vi "Edit_bad_calibration_coeff.vi"() -> ()   [LabVIEW 2010]
uses:
  Anemometry Sub Vis/Controls/File_Selector_Type.ctl
  Anemometry Sub Vis/Globals/Meas_global.vi
panel:
  out "index of element":i32
  out "bkgnd":string
  in  "Previous Choice":path
  in  "Search String":string
  in  "Boolean":bool
  in  "Pause Mode":enum16{"Continuous Running", "After Each File"}(ring)
  in  "At Dialog Prompt Post Process":T1
  out "Files Processed":i32(slide) scale=0.0..1.0
  in  "stop":bool
  out "Files To Process":path[](array[path])
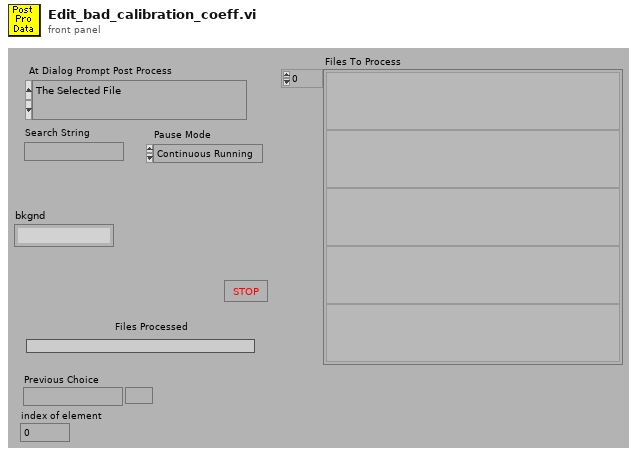
[diagram p1: front panel]
types:
  T1 = typedef "File_Selector_Type.ctl" = enum16{"The Selected File", "The Selected Folder", "Files containing the search string in the selected folder", "All files listed in selected file"}
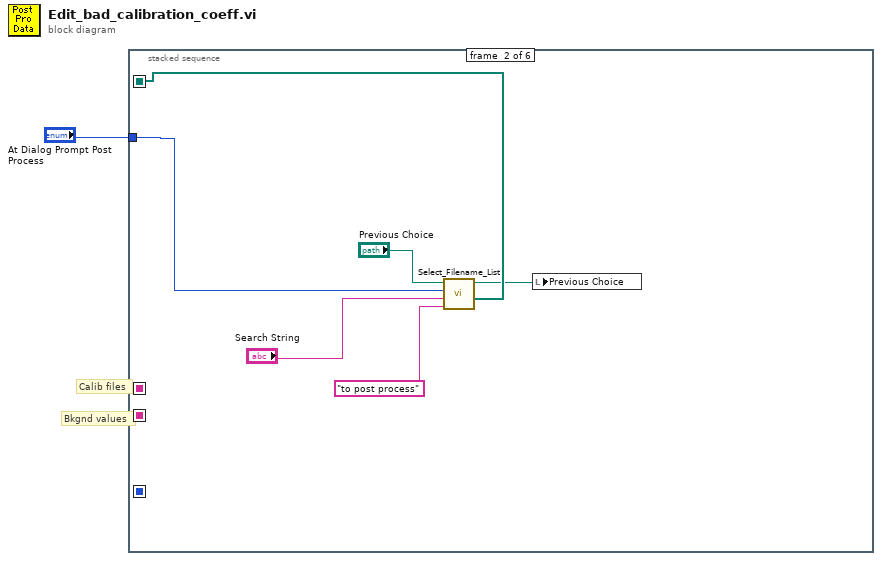
[diagram p0: block diagram]
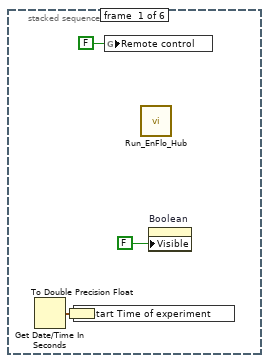
[diagram p2: hidden frame]
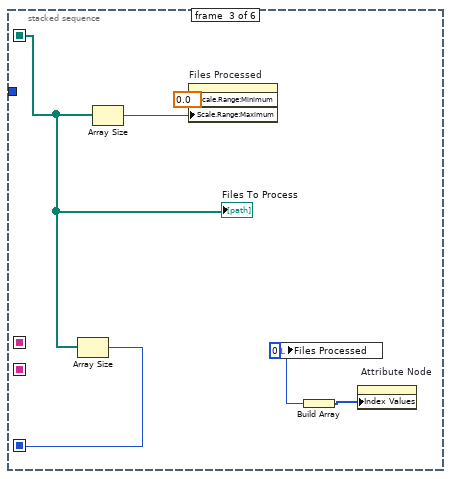
[diagram p3: hidden frame]
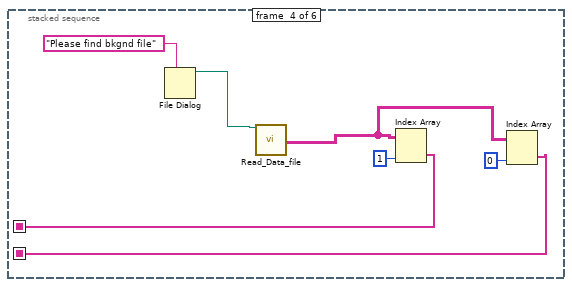
[diagram p4: hidden frame]
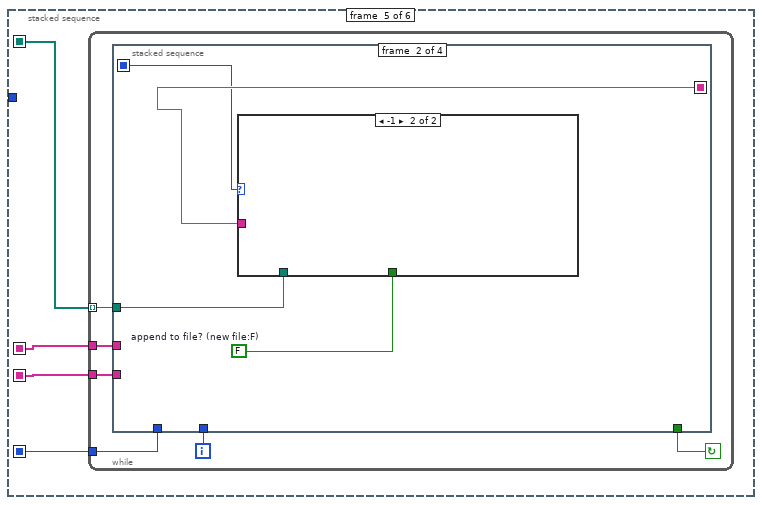
[diagram p5: hidden frame]
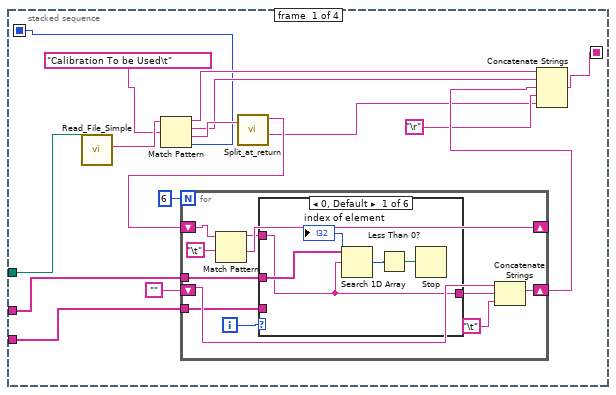
[diagram p6: hidden frame]
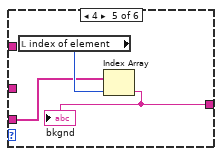
[diagram p10: hidden frame]
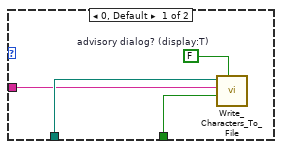
[diagram p12: hidden frame]
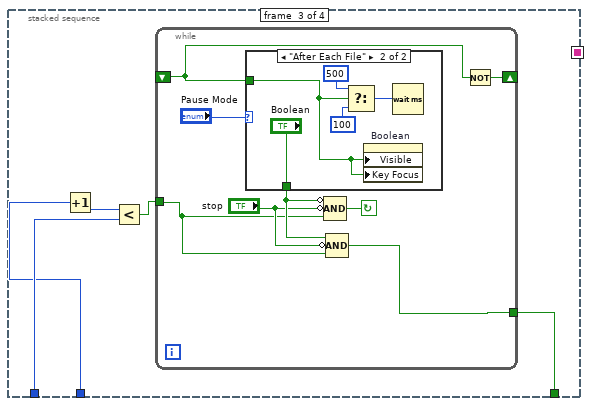
[diagram p13: hidden frame]
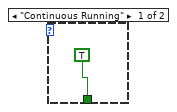
[diagram p14: hidden frame]
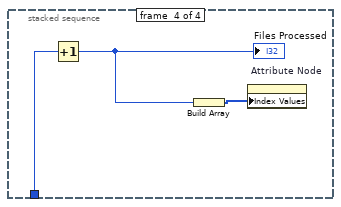
[diagram p15: hidden frame]
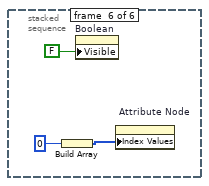
[diagram p16: hidden frame]
diagram:
  # "Bkgnd values"
  # "Calib files"
  n1 = stacked-sequence {
    seq-local: [_ _ w17 _ _ _] -> [_ _ _ _ w28 _]
    seq-local: [_ w10 _ _ _ _] -> [_ _ w12 _ w27 _]
    seq-local: [_ _ _ w21 _ _] -> [_ _ _ _ w26 _]
    seq-local: [_ _ _ w18 _ _] -> [_ _ _ _ w25 _]
    tunnel: "At Dialog Prompt Post Process" -> [_ w11 _ _ _ _]
    frame #0 {
      n2 = Get Date/Time In Seconds() -> (seconds since 1Jan1904=w2:timestamp)
      n3 = To Double Precision Float(number=w2) -> (double precision float=w3:dbl)
      n4 = global write "Meas_global.vi" "Start Time of experiment"(w3) -> ()
      n5 = global write "Meas_global.vi" "Remote control"(FALSE ("Remote control")) -> ()
      n6 = call "Run_EnFlo_Hub.vi"() -> ()  [unwired: 8 in]
      n7 = property on="Boolean" class="Bool"("Visible"=FALSE ("Write Attribute")) -> ()  [unwired: 2 in, 2 out]
    }
    frame #1 {
      n8 = call "Select_Filename_List.vi"("File Type"="to post process", "Search String"="Search String", "At Dialog Prompt Post Process"=w11, "Previous Choice"="Previous Choice") -> ("Selected files"=w10:path[], "Choosen path"=w6:path)  [unwired: 2 in, 1 out]
      n9 = local write "Previous Choice"(w6) -> ()
    }
    frame #2 {
      w13 = 0 ("Files Processed")
      n10 = Array Size(array=w12) -> (size(s)=w17:i32)
      n11 = Array Size(array=w12) -> (size(s)=w15:i32)
      n12 = property on="Files Processed" class="Slide (strict)"("Scale.Range:Minimum"=0.0 ("Write Attribute"), "Scale.Range:Maximum"=w15) -> ()  [unwired: 2 in, 2 out]
      n13 = local write "Files Processed"(w13) -> ()
      n14 = Build Array(w13) -> (w14:i32[])
      n15 = property on="Attribute Node" class="Arr (strict)"("Index Values"=w14) -> ()  [unwired: 2 in, 2 out]
      "Files To Process" <- w12
    }
    frame #3 {
      n16 = File Dialog(7:"Please find bkgnd file" ("prompt")) -> (3:w23:path)  [unwired: 6 in, 3 out]
      n17 = call "Read_Data_file.vi"("Results file"=w23) -> ("Channel Values Out"=w19:string[][])  [unwired: 9 in, 9 out]
      n18 = Index Array(array=w19, index (col)=1 ("disabled index (col)")) -> (element=w21:string[])  [unwired: 1 in]
      n19 = Index Array(array=w19, index (col)=0 ("disabled index (col)")) -> (element=w18:string[])  [unwired: 1 in]
    }
    frame #4 {
      n20 = while {
        tunnel: w27 -> [w31] mode=indexing
        tunnel: w28 -> [w34]
        tunnel: w26 -> [w30]
        tunnel: w25 -> [w29]
        i -> [w33]
        stop <- w32 continue-if-true
        n21 = stacked-sequence {
          seq-local: [w40 _ _ _] -> [_ w74 _ _]
          seq-local: [w35 _ _ _] -> [_ w73 _ _]
          tunnel: w31 -> [w50 w76 _ _]
          tunnel: w34 -> [_ _ w83 _]
          tunnel: w33 -> [_ _ w82 w101]
          tunnel: [_ _ w81 _] -> w32
          tunnel: w30 -> [w37 _ _ _]
          tunnel: w29 -> [w36 _ _ _]
          frame #0 {
            n22 = call "Read_File_Simple.vi"("Filename"=w50) -> ("string"=w47:string)  [unwired: 4 in, 5 out]
            n23 = Match Pattern(string=w47, regular expression="Calibration To be Used\t" ("Variable name")) -> (before substring=w43:string, match substring=w42:string, after substring=w45:string, offset past match=w35:i32)  [unwired: 1 in]
            n24 = call "Split_at_return.vi"("String"=w45) -> ("before substring"=w44:string, "after substring"=w38:string)  [unwired: 1 in, 2 out]
            n25 = for {
              N: 6 -> [_]
              shift-right: [w55] -> _
              shift-left: w44 -> [w60]
              shift-right: [w56] -> w41
              shift-left: "" -> [w58]
              tunnel: w37 -> [w52]
              tunnel: w36 -> [w51]
              i -> [w59]
              n26 = Match Pattern(string=w60, regular expression="\t") -> (before substring=w53:string, after substring=w55:string)  [unwired: 1 in, 2 out]
              n27 = case shown="0, Default" w59 {
                tunnel: [w64 w66 w67 w68 w69 w72] -> w54
                tunnel: w53 -> [w64 w66 w67 w68 _ w72]
                tunnel: w52 -> [w65 _ _ _ _ _]
                tunnel: w51 -> [_ _ _ _ w70 _]
                frame 0, Default {
                  n28 = Search 1D Array(1D array=w65, element=w64) -> (index of element=w63:i32)  [unwired: 1 in]
                  "index of element" <- w63
                  n29 = Less Than 0?(x=w63) -> (x < 0?=w62:bool)
                  n30 = Stop(stop? (T)=w62) -> ()
                }
                frame 1 {
                }
                frame 2 {
                }
                frame 3 {
                }
                frame 4 {
                  n31 = local read "index of element"() -> (w71:i32)
                  n32 = Index Array(array=w70, index=w71) -> (element=w69:string)
                  "bkgnd" <- w69
                }
                frame 5 {
                }
              }
              n33 = Concatenate Strings(w58, w54, "\t") -> (w56:string)
            }
            n34 = Concatenate Strings(w43, w42, w41, "\r", w38) -> (w40:string)
          }
          frame #1 {
            w75 = FALSE  # append to file? (new file:F)
            n35 = case shown="-1" w73 {
              tunnel: w76 -> [w80 _]
              tunnel: w75 -> [w78 _]
              tunnel: w74 -> [w77 _]
              frame 0, Default {
                w79 = FALSE  # advisory dialog? (display:T)
                n36 = call "Write_Characters_To_File.vi"("file path (dialog if empty)"=w80, "advisory dialog? (display:T)"=w79, "character string"=w77, "append to file? (new file:F)"=w78) -> ()  [unwired: 4 in, 1 out]
              }
              frame -1 {
              }
            }
          }
          frame #2 {
            n37 = Increment(x=w82) -> (x+1=w85:i32)
            n38 = Less?(x=w85, y=w83) -> (x < y?=w84:bool)
            n39 = while {
              shift-left: _ -> [w91]
              shift-right: [w92] -> _
              tunnel: [w86] -> w81
              tunnel: w84 -> [w87]
              stop <- w90 continue-if-true
              n40 = case shown="\"After Each File\"" "Pause Mode" {
                tunnel: [TRUE "Boolean"] -> w89
                tunnel: w91 -> [_ w98]
                frame "Continuous Running" {
                }
                frame "After Each File" {
                  n41 = Select(t=u32 500 ("milliseconds to wait"), s=w98, f=u32 100) -> (s? t:f=w95:u32)
                  n42 = property on="Boolean" class="Bool"("Visible"=w98, "Key Focus"=w98) -> ()  [unwired: 2 in, 2 out]
                  n43 = Wait (ms)(milliseconds to wait=w95) -> ()  [unwired: 1 out]
                }
              }
              n44 = Compound Arithmetic op=AND(invert w89, invert "stop", w87) -> (w90:bool)
              n45 = Compound Arithmetic op=AND(w89, invert "stop", w87) -> (w86:bool)
              n46 = Not(x=w91) -> (.not. x?=w92:bool)
            }
          }
          frame #3 {
            n47 = Increment(x=w101) -> (x+1=w100:i32)
            "Files Processed" <- w100
            n48 = Build Array(w100) -> (w102:i32[])
            n49 = property on="Attribute Node" class="Arr (strict)"("Index Values"=w102) -> ()  [unwired: 2 in, 2 out]
          }
        }
      }
    }
    frame #5 {
      n50 = Build Array(0) -> (w104:i32[])
      n51 = property on="Boolean" class="Bool"("Visible"=FALSE ("Write Attribute")) -> ()  [unwired: 2 in, 2 out]
      n52 = property on="Attribute Node" class="Arr (strict)"("Index Values"=w104) -> ()  [unwired: 2 in, 2 out]
    }
  }
